vi "Read Transient Data and Write to Shared Variable.vi"(8 "error in":errorcluster, 10 "Maximum Waveform Length":i32=10000) -> (0 "error out":errorcluster)   [LabVIEW 2017, in "DTACQ - Network Enabled Device Driver.lvlib"]
doc: "Downloads data from the device and publishes that data to shared variables"
uses:
  DTACQ - Network Enabled Device Driver.lvlib
  Communications/Typedefs/DTACQ Module Carrier Configuration--Cluster.ctl
  Communications/Typedefs/DTACQ Module Configuration--Cluster.ctl
  Communications/Typedefs/DTACQ Device Type--Enum.ctl
  Network Shared Variables/Typedefs/X and Y Variant Arrays--Cluster.ctl
  FGV Operaions--Enum.ctl
  Network Shared Variables/Shared Variables Library.lvlib
  Communications/Communications Library.lvlib
panel:
  in  "Carrier Configuration":T1={"Name"="Default Settings", "IP"="192.168.0.84", "Control Port"=4220, "Timeout (ms)"=2000, "Continuous Capture Port (Multiplexed)"=4210, "Start HIL Shot Port"=53999, "AWG Upload Port (Multiplexed)"=54201, "Download Captured Data Port (Multiplexed)"=53000, "Module Slots"=2, "Module Configurations"=[{"Name"="ACQ 425 ELF", "Position"="192.168.0.84", "Module Type"=enum."Analog In Module", "Control Port"=4221, "Timeout (ms)"=2000, "Channels"=16}, {"Name"="AO 424 ELF", "Position"="192.168.0.84", "Module Type"=enum."Analog Out Module", "Control Port"=4222, "Timeout (ms)"=2000, "Channels"=16}]}
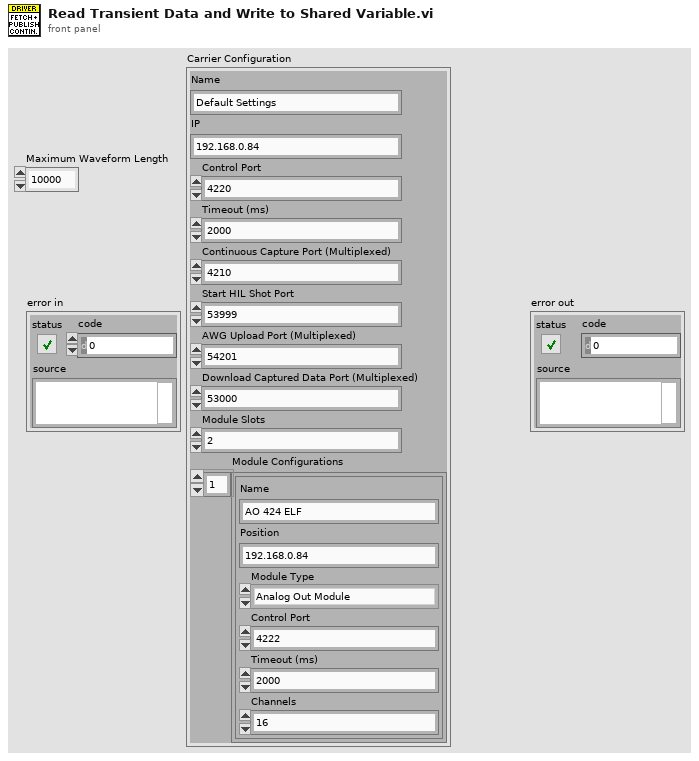
[diagram p1: front panel]
types:
  T1 = typedef "Communications Library.lvlib/DTACQ Module Carrier Configuration--Cluster.ctl" = cluster{"Name":string, "IP":string, "Control Port":i32, "Timeout (ms)":i32, "Continuous Capture Port (Multiplexed)":i32, "Start HIL Shot Port":i32, "AWG Upload Port (Multiplexed)":i32, "Download Captured Data Port (Multiplexed)":i32, "Module Slots":i32, "Module Configurations":T2[]}
  T2 = typedef "Communications Library.lvlib/DTACQ Module Configuration--Cluster.ctl" = cluster{"Name":string, "Position":string, "Module Type":T3, "Control Port":i32, "Timeout (ms)":i32, "Channels":i32}
  T3 = typedef "Communications Library.lvlib/DTACQ Device Type--Enum.ctl" = enum16{"Carrier", "Analog In Module", "Analog Out Module", "Generic Module"}
  T4 = typedef "DTACQ - Network Enabled Device Driver.lvlib/FGV Operaions--Enum.ctl" = enum16{"Get Driver Settings", "Set Driver Settings", "Search Variable Names", "Close Connections", "Open Connections", "Get Variable References", "Set Variable References", "Clear"}
  T5 = typedef "Shared Variables Library.lvlib/X and Y Variant Arrays--Cluster.ctl" = cluster{"X-Data":variant[], "Y-Data":variant[]}
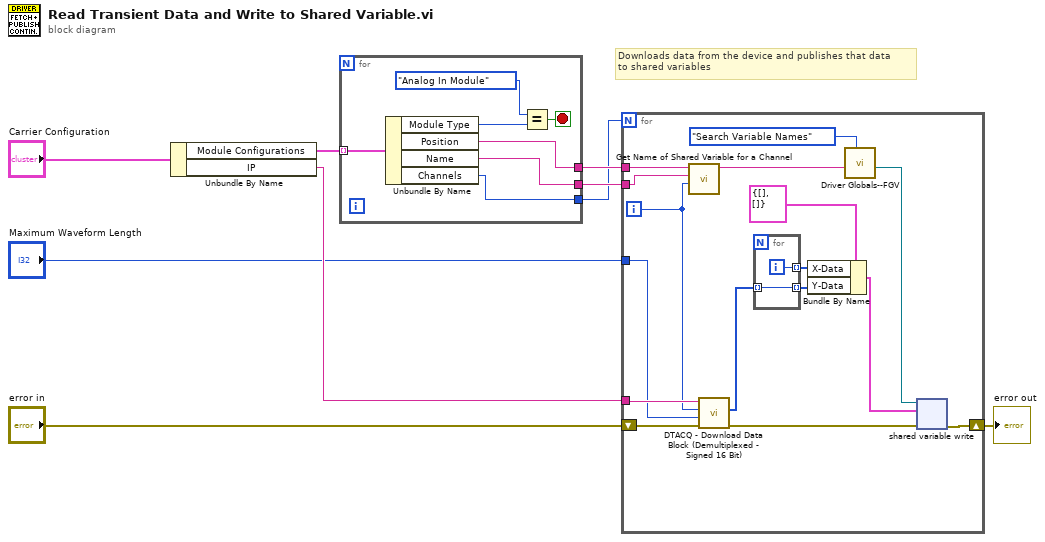
[diagram p0: block diagram]
diagram:
  # "Downloads data from the device and publishes that data\nto shared variables"
  n1 = Unbundle By Name("Carrier Configuration") -> ("Module Configurations"=w7:T2[], "IP"=w4:string)
  n2 = for {
    tunnel: w7 -> [w14] mode=indexing
    tunnel: [w12] -> w6
    tunnel: [w11] -> w5
    tunnel: [w10] -> w3
    stop <- w13 stop-if-true
    n3 = Unbundle By Name(w14) -> ("Module Type"=w16:T3, "Position"=w12:string, "Name"=w11:string, "Channels"=w10:i32)
    n4 = Equal?(x=DTACQ_Device_Type--Enum."Analog In Module", y=w16) -> (x = y?=w13:bool)
  }
  n5 = for {
    N: w3 -> [_]
    tunnel: w6 -> [w32]
    tunnel: w5 -> [w31]
    shift-right: [w25] -> w9
    shift-left: "error in" -> [w23]
    tunnel: w4 -> [w22]
    tunnel: "Maximum Waveform Length" -> [w18]
    i -> [w17]
    n6 = call "Get Name of Shared Variable for a Channel.vi"("Channel Number"=w17, "Module Name"=w31, "Module Position"=w32) -> ("Shared Variable Name"=w28:string)  [unwired: 8 in]
    n7 = call "DTACQ - Download Data Block (Demultiplexed - Signed 16 Bit).vi"("error in"=w23, "Maximum Number of Samples"=w18, "Channel Number"=w17, "Address"=w22) -> ("error out"=w24:errorcluster, "(Signed) 16 Bit Array"=w21:i16[])  [unwired: 5 in, 1 out]
    n8 = for {
      tunnel: [w34] -> w20 mode=indexing
      tunnel: w21 -> [w34] mode=indexing
      tunnel: [w33] -> w19 mode=indexing
      i -> [w33]
    }
    n9 = Bundle By Name(cluster=T5 {"X-Data"=[], "Y-Data"=[]} ("Data Cluster"), "X-Data"=w19, "Y-Data"=w20) -> (w26:T5)
    n10 = call "Driver Globals--FGV.vi"(7:FGV_Operaions--Enum."Search Variable Names", "Name"=w28) -> ("Searched Reference"=w27:refnum<k21>)  [unwired: 6 in, 3 out]
    n11 = shared-variable-write(w27, w24, w26) -> (w25:errorcluster)  [unwired: 1 out]
  }
  "error out" <- w9
